vi "log analysis_gps.vi"() -> ()   [LabVIEW 2019] (continued)
\t", "INSPVAXA,USB3,0,48.0,FINESTEERING,2107,282547.800,02000000,471d,15824;INS_ALIGNMENT_COMPLETE,INS_RTKFIXED,37.37036979022,126.72474424169,11.9829,22.3000,0.0059,0.0077,0.0009,-0.935404379,-0.556069366,17.549298346,0.2070,0.1677,0.2732,0.0344,0.0343,0.0312,0.0907,0.0906,5.0042,0f000005,0*a5f569c8\n\t", "INSPVAXA,USB3,0,52.0,FINESTEERING,2107,282548.300,02000000,471d,15824;INS_ALIGNMENT_COMPLETE,INS_RTKFIXED,37.37036979009,126.72474424298,11.9833,22.3000,0.0058,0.0072,0.0008,-0.938145117,-0.556054082,17.551756735,0.2062,0.1674,0.2718,0.0344,0.0343,0.0312,0.0907,0.0906,5.0051,0f000005,0*c2e33c02\n\t", "INSPVAXA,USB3,0,50.5,FINESTEERING,2107,282549.300,02000000,471d,15824;INS_ALIGNMENT_COMPLETE,INS_RTKFIXED,37.37036979437,126.72474424171,11.9842,22.3000,0.0072,0.0058,0.0011,-0.941172709,-0.557765925,17.557830544,0.2056,0.1673,0.2705,0.0344,0.0343,0.0312,0.0907,0.0905,5.0063,0f000005,0*401534f2\n\t", "INSPVAXA,USB3,0,50.5,FINESTEERING,2107,282549.800,02000000,471d,15824;INS_ALIGNMENT_COMPLETE,INS_RTKFIXED,37.37037057498,126.72474454669,11.9842,22.3000,0.3344,0.1212,-0.0021,-0.779908756,-0.829652021,16.234479944,0.2056,0.1673,0.2705,0.0344,0.0343,0.0312,0.0907,0.0905,5.0063,0f000005,0*992e23a9\n\t", "INSPVAXA,USB3,0,48.5,FINESTEERING,2107,282550.300,02000000,471d,15824;INS_ALIGNMENT_COMPLETE,INS_RTKFIXED,37.37037180552,126.72474490570,11.9839,22.3000,0.3136,0.0717,0.0047,-0.762896217,-1.138555506,11.977754851,0.2091,0.1720,0.2750,0.0478,0.0529,0.0400,0.0942,0.0940,5.0079,0f000001,0*abd47146\n\t", "INSPVAXA,USB3,0,48.5,FINESTEERING,2107,282550.800,02000000,471d,15824;INS_ALIGNMENT_COMPLETE,INS_RTKFIXED,37.37037314462,126.72474521124,11.9825,22.3000,0.2954,0.0405,-0.0041,-0.725905831,-1.406758813,6.746591451,0.2091,0.1720,0.2750,0.0478,0.0529,0.0400,0.0942,0.0940,5.0079,0f000001,0*61668905\n\t", "INSPVAXA,USB3,0,51.5,FINESTEERING,2107,282551.300,02000000,471d,15824;INS_ALIGNMENT_COMPLETE,INS_RTKFIXED,37.37037450282,126.72474542954,11.9799,22.3000,0.2952,0.0275,0.0043,-0.582539496,-1.551817939,1.239321391,0.2194,0.1781,0.2846,0.0602,0.0670,0.0471,0.0975,0.0974,5.0042,0f000001,0*c43f8c5d\n\t", "INSPVAXA,USB3,0,51.5,FINESTEERING,2107,282551.800,02000000,471d,15824;INS_ALIGNMENT_COMPLETE,INS_RTKFIXED,37.37037589392,126.72474545445,11.9759,22.3000,0.2950,0.0095,-0.0088,-0.557235878,-1.675921373,356.051789382,0.2194,0.1781,0.2846,0.0602,0.0670,0.0471,0.0975,0.0974,5.0042,0f000001,0*a284eeef\n\t", "INSPVAXA,USB3,0,51.0,FINESTEERING,2107,282552.300,02000000,471d,15824;INS_ALIGNMENT_COMPLETE,INS_RTKFIXED,37.37037725637,126.72474539414,11.9729,22.3000,0.3193,-0.0395,-0.0058,-0.358098572,-1.586037546,351.118490428,0.2390,0.1944,0.2996,0.0720,0.0761,0.0531,0.1006,0.1005,4.9843,0f000001,0*9b67c117\n\t", "INSPVAXA,USB3,0,51.0,FINESTEERING,2107,282552.800,02000000,471d,15824;INS_ALIGNMENT_COMPLETE,INS_RTKFIXED,37.37037867024,126.72474521498,11.9693,22.3000,0.3100,-0.0524,0.0074,-0.558642327,-1.723684038,345.940999200,0.2390,0.1944,0.2996,0.0720,0.0761,0.0531,0.1006,0.1005,4.9843,0f000001,0*b237e03e\n\t", "INSPVAXA,USB3,0,50.0,FINESTEERING,2107,282553.800,02000000,471d,15824;INS_ALIGNMENT_COMPLETE,INS_RTKFIXED,37.37038133440,126.72474444492,11.9605,22.3000,0.3081,-0.0778,-0.0137,-0.440969194,-1.715960461,335.579383056,0.2674,0.2182,0.3198,0.0835,0.0827,0.0582,0.1031,0.1033,4.9481,0f000001,0*e6869deb\n\t", "INSPVAXA,USB3,0,50.5,FINESTEERING,2107,282554.300,02000000,471d,15824;INS_ALIGNMENT_COMPLETE,INS_RTKFIXED,37.37038260490,126.72474387942,11.9550,22.3000,0.2856,-0.1157,-0.0141,-0.305818210,-1.684904810,330.613449941,0.3015,0.2424,0.3440,0.0942,0.0885,0.0625,0.1050,0.1055,4.9097,0f000001,0*224ecce4\n\t", "INSPVAXA,USB3,0,50.5,FINESTEERING,2107,282554.800,02000000,471d,15824;INS_ALIGNMENT_COMPLETE,INS_RTKFIXED,37.37038381003,126.72474321955,11.9506,22.3000,0.2827,-0.1438,-0.0083,-0.269920364,-1.529846026,325.201495362,0.3015,0.2424,0.3440,0.0942,0.0885,0.0625,0.1050,0.1055,4.9097,0f000001,0*3a829f91\n\t", "INSPVAXA,USB3,0,50.0,FINESTEERING,2107,282555.300,02000000,471d,15824;INS_ALIGNMENT_COMPLETE,INS_RTKFIXED,37.37038496801,126.72474241807,11.9455,22.3000,0.2577,-0.2027,-0.0062,-0.202108415,-1.553117740,320.165911198,0.3366,0.2625,0.3706,0.1033,0.0925,0.0661,0.1060,0.1070,4.8793,0f000001,0*992111cd\n\t", "INSPVAXA,USB3,0,50.0,FINESTEERING,2107,282555.800,02000000,471d,15824;INS_ALIGNMENT_COMPLETE,INS_RTKFIXED,37.37038604879,126.72474155018,11.9405,22.3000,0.2577,-0.1938,-0.0290,0.085654909,-1.443333237,315.847452046,0.3366,0.2625,0.3706,0.1033,0.0925,0.0661,0.1060,0.1070,4.8793,0f000001,0*a6375ebe\n\t", "INSPVAXA,USB3,0,47.0,FINESTEERING,2107,282556.300,02000000,471d,15824;INS_ALIGNMENT_COMPLETE,INS_RTKFIXED,37.37038704857,126.72474062241,11.9355,22.3000,0.2432,-0.1774,-0.0062,0.142331168,-1.481321498,311.639962663,0.3685,0.2772,0.3979,0.1103,0.0957,0.0690,0.1063,0.1076,4.8620,0f000001,0*be30efa1\n\t", "INSPVAXA,USB3,0,47.0,FINESTEERING,2107,282556.800,02000000,471d,15824;INS_ALIGNMENT_COMPLETE,INS_RTKFIXED,37.37038792888,126.72473964017,11.9328,22.3000,0.2236,-0.2049,0.0022,0.167042140,-1.399079221,308.149842307,0.3685,0.2772,0.3979,0.1103,0.0957,0.0690,0.1063,0.1076,4.8620,0f000001,0*295fc098\n\t", "INSPVAXA,USB3,0,49.5,FINESTEERING,2107,282557.300,02000000,471d,15824;INS_ALIGNMENT_COMPLETE,INS_RTKFIXED,37.37038876743,126.72473857634,11.9284,22.3000,0.2199,-0.2115,-0.0007,0.223675096,-1.209289977,305.425052983,0.3945,0.2871,0.4244,0.1154,0.0985,0.0713,0.1059,0.1076,4.8550,0f000001,0*37184781\n\t", "INSPVAXA,USB3,0,49.5,FINESTEERING,2107,282557.800,02000000,471d,15824;INS_ALIGNMENT_COMPLETE,INS_RTKFIXED,37.37038956876,126.72473745081,11.9243,22.3000,0.2096,-0.2177,-0.0233,0.358750528,-1.202788361,303.229385124,0.3945,0.2871,0.4244,0.1154,0.0985,0.0713,0.1059,0.1076,4.8550,0f000001,0*8c1e375a\n\t", "INSPVAXA,USB3,0,50.5,FINESTEERING,2107,282558.300,02000000,471d,15824;INS_ALIGNMENT_COMPLETE,INS_RTKFIXED,37.37039033864,126.72473628263,11.9208,22.3000,0.2004,-0.2164,-0.0069,0.499556511,-1.306604746,301.526266622,0.4138,0.2933,0.4487,0.1187,0.1006,0.0729,0.1051,0.1069,4.8540,0f000001,0*451656bf\n\t", "INSPVAXA,USB3,0,50.5,FINESTEERING,2107,282558.800,02000000,471d,15824;INS_ALIGNMENT_COMPLETE,INS_RTKFIXED,37.37039107336,126.72473508379,11.9182,22.3000,0.1823,-0.2245,-0.0036,0.428634950,-1.459936721,300.166492995,0.4138,0.2933,0.4487,0.1187,0.1006,0.0729,0.1051,0.1069,4.8540,0f000001,0*b88ea368\n\t", "INSPVAXA,USB3,0,48.0,FINESTEERING,2107,282559.300,02000000,471d,15824;INS_ALIGNMENT_COMPLETE,INS_RTKFIXED,37.37039179926,126.72473381878,11.9163,22.3000,0.1950,-0.2202,-0.0095,0.298148012,-1.385671812,299.213023137,0.4272,0.2974,0.4700,0.1208,0.1020,0.0740,0.1041,0.1060,4.8546,0f000001,0*f3b6d2c4\n\t", "INSPVAXA,USB3,0,48.0,FINESTEERING,2107,282559.800,02000000,471d,15824;INS_ALIGNMENT_COMPLETE,INS_RTKFIXED,37.37039251718,126.72473255012,11.9132,22.3000,0.1990,-0.2202,-0.0184,0.279170037,-1.304746130,298.607357050,0.4272,0.2974,0.4700,0.1208,0.1020,0.0740,0.1041,0.1060,4.8546,0f000001,0*fce9781a\n\t", "DUALANTENNAHEADINGA,USB3,0,49.0,FINESTEERING,2107,282560.300,02000000,d426,15824;SOL_COMPUTED,L1_FLOAT,-1.000000000,246.253692627,40.984443665,0.0,360.000000000,180.000000000,\"631T\",16,4,4,4,04,00,20,00*676df0ad\n\t", "INSPVAXA,USB3,0,49.0,FINESTEERING,2107,282560.800,02000000,471d,15824;INS_ALIGNMENT_COMPLETE,INS_RTKFIXED,37.37039395485,126.72472993141,11.9024,22.3000,0.2031,-0.2330,-0.0176,0.316707422,-1.216731962,298.161405387,0.4358,0.3002,0.4880,0.1220,0.1029,0.0748,0.1029,0.1049,4.8545,0f000001,0*df5ab1e4\n\t", "DUALANTENNAHEADINGA,USB3,0,50.5,FINESTEERING,2107,282561.300,02000000,d426,15824;SOL_COMPUTED,L1_FLOAT,-1.000000000,334.919982910,-70.914154053,0.0,360.000000000,180.000000000,\"631T\",14,4,4,4,04,00,20,00*464ca699\n\t", "INSPVAXA,USB3,0,50.5,FINESTEERING,2107,282561.800,02000000,471d,15824;INS_ALIGNMENT_COMPLETE,INS_RTKFIXED,37.37039536755,126.72472721872,11.8937,22.3000,0.2015,-0.2233,-0.0217,0.095358091,-1.276712032,298.220729276,0.4412,0.3019,0.5026,0.1224,0.1030,0.0752,0.1017,0.1038,4.8530,0f000001,0*c4564f75\n\t", "DUALANTENNAHEADINGA,USB3,0,50.0,FINESTEERING,2107,282562.300,02000000,d426,15824;SOL_COMPUTED,L1_FLOAT,-1.000000000,248.535232544,17.692501068,0.0,360.000000000,180.000000000,\"631T\",15,4,4,4,04,00,20,00*bc5c3482\n\t", "INSPVAXA,USB3,0,50.0,FINESTEERING,2107,282562.800,02000000,471d,15824;INS_ALIGNMENT_COMPLETE,INS_RTKFIXED,37.37039678441,126.72472449457,11.8837,22.3000,0.2087,-0.2358,-0.0215,0.255454294,-1.083158063,298.402079920,0.4444,0.3029,0.5140,0.1223,0.1022,0.0754,0.1006,0.1028,4.8501,0f000001,0*9eae090a\n\t", "DUALANTENNAHEADINGA,USB3,0,51.0,FINESTEERING,2107,282563.300,02000000,d426,15824;SOL_COMPUTED,L1_FLOAT,-1.000000000,237.849975586,47.216407776,0.0,360.000000000,180.000000000,\"631T\",15,4,4,4,04,00,20,00*b09d8761\n\t", "DUALANTENNAHEADINGA,USB3,0,51.0,FINESTEERING,2107,282563.800,02000000,d426,15824;SOL_COMPUTED,L1_FLOAT,-1.000000000,239.350723267,46.591415405,0.0,360.000000000,180.000000000,\"631T\",14,4,4,4,04,00,20,00*f242e7bf\n\t", "DUALANTENNAHEADINGA,USB3,0,51.0,FINESTEERING,2107,282564.300,02000000,d426,15824;SOL_COMPUTED,L1_FLOAT,-1.000000000,238.787353516,46.982643127,0.0,360.000000000,180.000000000,\"631T\",14,4,4,4,04,00,20,00*054ac6ab\n\t", "DUALANTENNAHEADINGA,USB3,0,51.0,FINESTEERING,2107,282564.800,02000000,d426,15824;SOL_COMPUTED,L1_FLOAT,-1.000000000,245.656951904,39.742870331,0.0,360.000000000,180.000000000,\"631T\",14,4,4,4,04,00,20,00*f11cb885\n\t", "DUALANTENNAHEADINGA,USB3,0,52.0,FINESTEERING,2107,282565.300,02000000,d426,15824;SOL_COMPUTED,L1_FLOAT,-1.000000000,248.154891968,40.657573700,0.0,360.000000000,180.000000000,\"631T\",14,4,4,4,04,00,20,00*20192c08\n\t", "INSPVAXA,USB3,0,52.0,FINESTEERING,2107,282565.800,02000000,471d,15824;INS_ALIGNMENT_COMPLETE,INS_RTKFIXED,37.37040119345,126.72471623377,11.8630,22.3000,0.2075,-0.2604,-0.0264,0.476736901,-1.637367273,299.264508322,0.4468,0.3026,0.5333,0.1200,0.0984,0.0755,0.0985,0.1009,4.8387,0f000001,0*ff25f4bc\n\t", "INSPVAXA,USB3,0,51.5,FINESTEERING,2107,282566.300,02000000,471d,15824;INS_ALIGNMENT_COMPLETE,INS_RTKFIXED,37.37040195558,126.72471483727,11.8592,22.3000,0.1958,-0.2436,-0.0278,0.510354865,-1.544191392,299.414254294,0.4462,0.3017,0.5364,0.1190,0.0970,0.0755,0.0983,0.1007,4.8363,0f000001,0*b461588d\n\t", "INSPVAXA,USB3,0,51.5,FINESTEERING,2107,282566.800,02000000,471d,15824;INS_ALIGNMENT_COMPLETE,INS_RTKFIXED,37.37040269281,126.72471352564,11.8555,22.3000,0.1908,-0.2417,-0.0283,0.566870659,-1.494613883,299.549327154,0.4462,0.3017,0.5364,0.1190,0.0970,0.0755,0.0983,0.1007,4.8363,0f000001,0*0dca09ad\n\t", "DUALANTENNAHEADINGA,USB3,0,48.5,FINESTEERING,2107,282567.300,02000000,d426,15824;SOL_COMPUTED,L1_FLOAT,-1.000000000,255.600921631,36.764995575,0.0,360.000000000,180.000000000,\"631T\",14,4,4,4,04,00,20,00*5c98ac44\n\t", "DUALANTENNAHEADINGA,USB3,0,48.5,FINESTEERING,2107,282567.800,02000000,d426,15824;SOL_COMPUTED,L1_FLOAT,-1.000000000,256.974517822,34.665092468,0.0,360.000000000,180.000000000,\"631T\",13,4,4,4,04,00,20,00*958b7579\n\t", "DUALANTENNAHEADINGA,USB3,0,47.5,FINESTEERING,2107,282568.300,02000000,d426,15824;SOL_COMPUTED,L1_FLOAT,-1.000000000,267.947265625,0.986307323,0.0,360.000000000,180.000000000,\"631T\",15,4,4,4,04,00,20,00*84956e00\n\t", "DUALANTENNAHEADINGA,USB3,0,47.5,FINESTEERING,2107,282568.800,02000000,d426,15824;SOL_COMPUTED,L1_FLOAT,-1.000000000,262.026367188,14.068168640,0.0,360.000000000,180.000000000,\"631T\",16,4,4,4,04,00,20,00*8f55d343\n\t", "DUALANTENNAHEADINGA,USB3,0,50.0,FINESTEERING,2107,282569.300,02000000,d426,15824;SOL_COMPUTED,L1_FLOAT,-1.000000000,247.101364136,35.273887634,0.0,360.000000000,180.000000000,\"631T\",16,4,4,3,04,00,20,00*a64cde4f\n\t", "DUALANTENNAHEADINGA,USB3,0,50.0,FINESTEERING,2107,282569.800,02000000,d426,15824;SOL_COMPUTED,L1_FLOAT,-1.000000000,275.467193604,-13.373962402,0.0,360.000000000,180.000000000,\"631T\",15,4,4,4,04,00,20,00*431901e2\n\t", "DUALANTENNAHEADINGA,USB3,0,51.0,FINESTEERING,2107,282570.300,02000000,d426,15824;SOL_COMPUTED,L1_FLOAT,-1.000000000,299.108795166,-43.822387695,0.0,360.000000000,180.000000000,\"631T\",15,4,4,4,04,00,20,00*983d1a38\n\t", "DUALANTENNAHEADINGA,USB3,0,51.0,FINESTEERING,2107,282570.800,02000000,d426,15824;SOL_COMPUTED,L1_FLOAT,-1.000000000,300.479248047,-46.014068604,0.0,360.000000000,180.000000000,\"631T\",16,4,4,4,04,00,20,00*471f7ae7\n\t", "DUALANTENNAHEADINGA,USB3,0,50.5,FINESTEERING,2107,282571.300,02000000,d426,15824;SOL_COMPUTED,L1_FLOAT,-1.000000000,281.970092773,-22.784423828,0.0,360.000000000,180.000000000,\"631T\",16,4,4,4,04,00,20,00*6e1b1745\n\t", "DUALANTENNAHEADINGA,USB3,0,50.5,FINESTEERING,2107,282571.800,02000000,d426,15824;SOL_COMPUTED,L1_FLOAT,-1.000000000,280.621307373,-20.287109375,0.0,360.000000000,180.000000000,\"631T\",17,4,4,4,04,00,20,00*f2e1552e\n\t", "DUALANTENNAHEADINGA,USB3,0,50.5,FINESTEERING,2107,282572.300,02000000,d426,15824;SOL_COMPUTED,L1_FLOAT,-1.000000000,248.617050171,42.773250580,0.0,360.000000000,180.000000000,\"631T\",14,4,4,4,04,00,20,00*4f7db08e\n\t", "DUALANTENNAHEADINGA,USB3,0,50.5,FINESTEERING,2107,282572.800,02000000,d426,15824;SOL_COMPUTED,L1_FLOAT,-1.000000000,246.696640015,43.920532227,0.0,360.000000000,180.000000000,\"631T\",15,4,4,4,04,00,20,00*5d650678\n\t", "DUALANTENNAHEADINGA,USB3,0,47.0,FINESTEERING,2107,282573.300,02000000,d426,15824;SOL_COMPUTED,L1_FLOAT,-1.000000000,245.228240967,45.089698792,0.0,360.000000000,180.000000000,\"631T\",15,6,6,6,04,00,20,20*cc0e41c2\n\t", "DUALANTENNAHEADINGA,USB3,0,47.0,FINESTEERING,2107,282573.800,02000000,d426,15824;SOL_COMPUTED,L1_FLOAT,-1.000000000,244.818725586,44.919303894,0.0,360.000000000,180.000000000,\"631T\",15,6,6,6,04,00,20,20*3059716a\n\t", "DUALANTENNAHEADINGA,USB3,0,50.0,FINESTEERING,2107,282574.300,02000000,d426,15824;SOL_COMPUTED,L1_FLOAT,-1.000000000,234.880477905,50.460414886,0.0,146.039688110,120.522598267,\"631T\",15,6,6,6,04,00,20,20*c87e4a6e\n\t", "DUALANTENNAHEADINGA,USB3,0,50.0,FINESTEERING,2107,282574.800,02000000,d426,15824;SOL_COMPUTED,L1_FLOAT,-1.000000000,234.896896362,50.646526337,0.0,146.141387939,119.189933777,\"631T\",17,6,6,6,04,00,20,20*6b091558\n\t", "DUALANTENNAHEADINGA,USB3,0,47.0,FINESTEERING,2107,282575.300,02000000,d426,15824;SOL_COMPUTED,L1_FLOAT,-1.000000000,247.052993774,4.654780388,0.0,360.000000000,180.000000000,\"631T\",15,6,6,6,04,00,20,20*6353fb30\n\t", "DUALANTENNAHEADINGA,USB3,0,47.0,FINESTEERING,2107,282575.800,02000000,d426,15824;SOL_COMPUTED,L1_FLOAT,-1.000000000,247.398025513,2.300915241,0.0,360.000000000,180.000000000,\"631T\",16,6,6,6,04,00,20,20*f5a4c1cb\n\t", "DUALANTENNAHEADINGA,USB3,0,49.5,FINESTEERING,2107,282577.300,02000000,d426,15824;SOL_COMPUTED,L1_FLOAT,-1.000000000,245.373901367,33.916652679,0.0,360.000000000,180.000000000,\"631T\",14,4,4,4,04,00,20,00*102f57bf\n\t", "DUALANTENNAHEADINGA,USB3,0,49.5,FINESTEERING,2107,282577.800,02000000,d426,15824;SOL_COMPUTED,L1_FLOAT,-1.000000000,248.600692749,29.202283859,0.0,360.000000000,180.000000000,\"631T\",15,4,4,3,04,00,20,00*eaef8a59\n\t", "DUALANTENNAHEADINGA,USB3,0,50.0,FINESTEERING,2107,282578.300,02000000,d426,15824;SOL_COMPUTED,L1_FLOAT,-1.000000000,273.737609863,2.134390354,0.0,360.000000000,180.000000000,\"631T\",15,4,4,4,04,00,20,00*8bcfc7c6\n\t", "INSPVAXA,USB3,0,51.0,FINESTEERING,2107,282579.350,02000000,471d,15824;INS_ALIGNMENT_COMPLETE,INS_RTKFIXED,37.37041740707,126.72467743060,11.7862,22.3000,0.1031,-0.2921,-0.0179,0.173397794,-1.623675165,282.783174290,0.4573,0.2990,0.5534,0.1157,0.0933,0.0771,0.0996,0.1047,4.8395,0f000001,0*3f071db4\n\t", "DUALANTENNAHEADINGA,USB3,0,51.0,FINESTEERING,2107,282579.800,02000000,d426,15824;SOL_COMPUTED,L1_FLOAT,-1.000000000,253.552474976,36.318763733,0.0,360.000000000,180.000000000,\"631T\",12,4,4,4,04,00,20,00*83b3b49e\n\t", "DUALANTENNAHEADINGA,USB3,0,48.0,FINESTEERING,2107,282580.300,02000000,d426,15824;SOL_COMPUTED,L1_FLOAT,-1.000000000,276.287109375,16.184204102,0.0,360.000000000,180.000000000,\"631T\",13,4,4,4,04,00,20,00*58df2e4e\n\t", "INSPVAXA,USB3,0,48.0,FINESTEERING,2107,282580.850,02000000,471d,15824;INS_ALIGNMENT_COMPLETE,INS_RTKFIXED,37.37041861647,126.72467286120,11.7829,22.3000,0.1085,-0.2996,-0.0146,0.381599119,-1.778654518,281.769285798,0.4580,0.2991,0.5538,0.1158,0.0932,0.0771,0.0996,0.1049,4.8397,0f000001,0*ecbe1c22\n\t", "DUALANTENNAHEADINGA,USB3,0,49.0,FINESTEERING,2107,282581.800,02000000,d426,15824;SOL_COMPUTED,L1_FLOAT,-1.000000000,244.951904297,46.151142120,0.0,329.327331543,180.000000000,\"631T\",12,4,4,4,04,00,20,00*1c1834ad\n\t", "INSPVAXA,USB3,0,49.5,FINESTEERING,2107,282582.850,02000000,471d,15824;INS_ALIGNMENT_COMPLETE,INS_RTKFIXED,37.37042013529,126.72466675412,11.7738,22.3000,0.0889,-0.2912,-0.0157,0.137018151,-1.334468427,280.534881050,0.4569,0.2986,0.5535,0.1156,0.0931,0.0772,0.0995,0.1050,4.8407,0f000001,0*4cc88e7a\n\t", "DUALANTENNAHEADINGA,USB3,0,50.0,FINESTEERING,2107,282583.800,02000000,d426,15824;SOL_COMPUTED,L1_FLOAT,-1.000000000,298.425811768,-39.243469238,0.0,360.000000000,180.000000000,\"631T\",12,4,4,4,04,00,20,00*99234be7\n\t", "INSPVAXA,USB3,0,50.0,FINESTEERING,2107,282584.350,02000000,471d,15824;INS_ALIGNMENT_COMPLETE,INS_RTKFIXED,37.37042121578,126.72466218098,11.7682,22.3000,0.0908,-0.2905,-0.0097,0.228953863,-0.969786949,279.904204523,0.4542,0.2977,0.5520,0.1156,0.0930,0.0771,0.0995,0.1050,4.8423,0f000001,0*25d05607\n\t", "DUALANTENNAHEADINGA,USB3,0,50.0,FINESTEERING,2107,282584.800,02000000,d426,15824;SOL_COMPUTED,L1_FLOAT,-1.000000000,317.813751221,-55.080688477,0.0,360.000000000,180.000000000,\"631T\",14,4,4,4,04,00,20,00*482add9e\n\t", "DUALANTENNAHEADINGA,USB3,0,47.5,FINESTEERING,2107,282585.300,02008000,d426,15824;SOL_COMPUTED,L1_FLOAT,-1.000000000,279.031005859,-12.437835693,0.0,360.000000000,180.000000000,\"631T\",14,4,4,4,04,00,20,00*e33ff00b\n\t", "DUALANTENNAHEADINGA,USB3,0,47.5,FINESTEERING,2107,282585.800,02008000,d426,15824;SOL_COMPUTED,L1_FLOAT,-1.000000000,288.534484863,-28.210021973,0.0,360.000000000,180.000000000,\"631T\",14,4,4,4,04,00,20,00*75d90e5f\n\t", "DUALANTENNAHEADINGA,USB3,0,47.0,FINESTEERING,2107,282586.800,02008000,d426,15824;SOL_COMPUTED,L1_FLOAT,-1.000000000,299.638763428,-44.873535156,0.0,360.000000000,180.000000000,\"631T\",12,4,4,4,04,00,20,00*8433efc6\n\t", "DUALANTENNAHEADINGA,USB3,0,51.0,FINESTEERING,2107,282587.800,02008000,d426,15824;SOL_COMPUTED,L1_FLOAT,-1.000000000,274.837402344,7.455324173,0.0,360.000000000,180.000000000,\"631T\",12,4,4,4,04,00,20,00*d357c890\n\t", "INSPVAXA,USB3,0,53.0,FINESTEERING,2107,282588.350,02008000,471d,15824;INS_ALIGNMENT_COMPLETE,INS_RTKFIXED,37.37042392170,126.72464987629,11.7560,22.3000,0.0923,-0.2810,-0.0093,0.030566631,-0.932089530,279.991317390,0.4489,0.2966,0.5498,0.1150,0.0928,0.0771,0.0995,0.1049,4.8445,0f000001,0*cf0f29b3\n\t", "DUALANTENNAHEADINGA,USB3,0,53.0,FINESTEERING,2107,282588.800,02008000,d426,15824;SOL_COMPUTED,L1_FLOAT,-1.000000000,322.314697266,-55.526092529,0.0,360.000000000,180.000000000,\"631T\",12,4,4,4,04,00,20,00*c23a8009\n\t", "INSPVAXA,USB3,0,51.5,FINESTEERING,2107,282589.350,02000000,471d,15824;INS_ALIGNMENT_COMPLETE,INS_RTKFIXED,37.37042463832,126.72464679942,11.7536,22.3000,0.0961,-0.3116,-0.0160,0.320803902,-1.173970058,280.179307501,0.4487,0.2962,0.5495,0.1150,0.0928,0.0771,0.0995,0.1049,4.8450,0f000001,0*5f568f32\n\t", "INSPVAXA,USB3,0,51.5,FINESTEERING,2107,282589.850,02000000,471d,15824;INS_ALIGNMENT_COMPLETE,INS_RTKFIXED,37.37042500999,126.72464523335,11.7530,22.3000,0.0866,-0.2870,-0.0118,0.410270840,-1.158910418,280.360984304,0.4487,0.2962,0.5495,0.1150,0.0928,0.0771,0.0995,0.1049,4.8450,0f000001,0*cae4522e\n\t", "DUALANTENNAHEADINGA,USB3,0,50.5,FINESTEERING,2107,282590.300,02000000,d426,15824;INSUFFICIENT_OBS,NONE,-1.000000000,0.000000000,0.000000000,0.0,0.000000000,0.000000000,\"631T\",14,3,3,3,04,00,20,00*40a503c4\n\t", "INSPVAXA,USB3,0,49.0,FINESTEERING,2107,282591.350,02000000,471d,15824;INS_ALIGNMENT_COMPLETE,INS_RTKFIXED,37.37042612746,126.72464043128,11.7509,22.3000,0.1112,-0.3046,-0.0107,0.438593312,-1.353837387,280.922848312,0.4465,0.2958,0.5485,0.1145,0.0928,0.0771,0.0995,0.1048,4.8451,0f000001,0*466c5cb5\n\t", "INSPVAXA,USB3,0,48.0,FINESTEERING,2107,282592.350,02000000,471d,15824;INS_ALIGNMENT_COMPLETE,INS_RTKFIXED,37.37042693515,126.72463721970,11.7478,22.3000,0.1134,-0.2841,-0.0136,0.495116506,-1.748021922,281.445386324,0.4458,0.2955,0.5484,0.1143,0.0927,0.0771,0.0996,0.1048,4.8449,0f000001,0*7d422fc0\n\t", "INSPVAXA,USB3,0,51.5,FINESTEERING,2107,282593.350,02000000,471d,15824;INS_ALIGNMENT_COMPLETE,INS_RTKFIXED,37.37042777147,126.72463409939,11.7416,22.3000,0.1053,-0.2907,-0.0160,0.642644908,-1.933701573,282.530113202,0.4438,0.2953,0.5477,0.1141,0.0928,0.0771,0.0997,0.1048,4.8448,0f000001,0*602d795b\n\t", "INSPVAXA,USB3,0,51.5,FINESTEERING,2107,282593.850,02000000,471d,15824;INS_ALIGNMENT_COMPLETE,INS_RTKFIXED,37.37042819780,126.72463255781,11.7390,22.3000,0.0952,-0.2916,-0.0106,0.650646949,-1.972506612,283.259305122,0.4438,0.2953,0.5477,0.1141,0.0928,0.0771,0.0997,0.1048,4.8448,0f000001,0*d7827024\n\t", "INSPVAXA,USB3,0,49.5,FINESTEERING,2107,282594.350,02000000,471d,15824;INS_ALIGNMENT_COMPLETE,INS_RTKFIXED,37.37042864678,126.72463101246,11.7344,22.3000,0.0979,-0.2869,-0.0099,0.556878145,-1.878860029,284.055732763,0.4423,0.2949,0.5470,0.1139,0.0928,0.0770,0.0997,0.1048,4.8442,0f000001,0*f7248edf\n\t", "INSPVAXA,USB3,0,49.5,FINESTEERING,2107,282594.850,02000000,471d,15824;INS_ALIGNMENT_COMPLETE,INS_RTKFIXED,37.37042912060,126.72462947652,11.7289,22.3000,0.1303,-0.2985,-0.0065,0.456318200,-1.931761270,284.972124281,0.4423,0.2949,0.5470,0.1139,0.0928,0.0770,0.0997,0.1048,4.8442,0f000001,0*61f64e67\n\t", "INSPVAXA,USB3,0,48.5,FINESTEERING,2107,282595.350,02000000,471d,15824;INS_ALIGNMENT_COMPLETE,INS_RTKFIXED,37.37042961366,126.72462798098,11.7236,22.3000,0.1497,-0.2970,-0.0149,0.418327229,-1.868019582,285.752151928,0.4414,0.2947,0.5465,0.1139,0.0925,0.0770,0.0998,0.1049,4.8430,0f000001,0*1a617db7\n\t", "INSPVAXA,USB3,0,48.5,FINESTEERING,2107,282595.850,02000000,471d,15824;INS_ALIGNMENT_COMPLETE,INS_RTKFIXED,37.37043014219,126.72462646518,11.7180,22.3000,0.1392,-0.2900,-0.0231,0.427669167,-1.922456438,286.476446001,0.4414,0.2947,0.5465,0.1139,0.0925,0.0770,0.0998,0.1049,4.8430,0f000001,0*1a66d065\n\t", "INSPVAXA,USB3,0,50.5,FINESTEERING,2107,282596.350,02000000,471d,15824;INS_ALIGNMENT_COMPLETE,INS_RTKFIXED,37.37043069447,126.72462494509,11.7122,22.3000,0.1569,-0.2925,-0.0148,0.456002187,-2.188056466,287.205419298,0.4412,0.2946,0.5461,0.1139,0.0925,0.0770,0.0999,0.1050,4.8425,0f000001,0*15a09225\n\t", "INSPVAXA,USB3,0,50.5,FINESTEERING,2107,282596.850,02000000,471d,15824;INS_ALIGNMENT_COMPLETE,INS_RTKFIXED,37.37043125589,126.72462344785,11.7060,22.3000,0.1402,-0.2734,-0.0172,0.395468070,-2.411480135,287.743907623,0.4412,0.2946,0.5461,0.1139,0.0925,0.0770,0.0999,0.1050,4.8425,0f000001,0*9ae986ea\n\t", "INSPVAXA,USB3,0,49.0,FINESTEERING,2107,282597.350,02000000,471d,15824;INS_ALIGNMENT_COMPLETE,INS_RTKFIXED,37.37043180809,126.72462197460,11.7004,22.3000,0.1451,-0.2798,-0.0240,0.082189404,-2.342857619,288.211463548,0.4406,0.2943,0.5456,0.1138,0.0925,0.0770,0.1000,0.1050,4.8425,0f000001,0*a4baef99\n\t", "INSPVAXA,USB3,0,47.0,FINESTEERING,2107,282598.350,02000000,471d,15824;INS_ALIGNMENT_COMPLETE,INS_RTKFIXED,37.37043296335,126.72461906573,11.6872,22.3000,0.1639,-0.2709,-0.0144,0.075715172,-2.060890876,288.886128801,0.4401,0.2937,0.5452,0.1138,0.0925,0.0770,0.1001,0.1051,4.8435,0f000001,0*53c08aab\n\t", "INSPVAXA,USB3,0,47.0,FINESTEERING,2107,282598.850,02000000,471d,15824;INS_ALIGNMENT_COMPLETE,INS_RTKFIXED,37.37043354014,126.72461760390,11.6788,22.3000,0.1599,-0.2669,-0.0128,0.049311349,-2.026534390,289.114340802,0.4401,0.2937,0.5452,0.1138,0.0925,0.0770,0.1001,0.1051,4.8435,0f000001,0*6b176d5a\n\t", "INSPVAXA,USB3,0,48.5,FINESTEERING,2107,282599.350,02000000,471d,15824;INS_ALIGNMENT_COMPLETE,INS_RTKFIXED,37.37043410493,126.72461616545,11.6719,22.3000,0.1624,-0.2885,-0.0138,-0.156644949,-2.114929380,289.341942256,0.4397,0.2935,0.5448,0.1139,0.0926,0.0770,0.1001,0.1052,4.8449,0f000001,0*992413bc\n\t", "INSPVAXA,USB3,0,48.5,FINESTEERING,2107,282599.850,02000000,471d,15824;INS_ALIGNMENT_COMPLETE,INS_RTKFIXED,37.37043467790,126.72461472498,11.6664,22.3000,0.1607,-0.2703,-0.0125,-0.362948004,-2.133534264,289.548423016,0.4397,0.2935,0.5448,0.1139,0.0926,0.0770,0.1001,0.1052,4.8449,0f000001,0*c10a254e\n\t", "INSPVAXA,USB3,0,49.5,FINESTEERING,2107,282600.350,02000000,471d,15824;INS_ALIGNMENT_COMPLETE,INS_RTKFIXED,37.37043525953,126.72461325909,11.6615,22.3000,0.1615,-0.2803,-0.0148,-0.471431775,-2.267846962,289.732073791,0.4392,0.2934,0.5443,0.1138,0.0928,0.0769,0.1001,0.1052,4.8460,0f000001,0*36a380c0\n\t", "INSPVAXA,USB3,0,49.5,FINESTEERING,2107,282600.850,02000000,471d,15824;INS_ALIGNMENT_COMPLETE,INS_RTKFIXED,37.37043586783,126.72461175288,11.6568,22.3000,0.1684,-0.2866,-0.0132,-0.451303759,-2.269558677,289.856432048,0.4392,0.2934,0.5443,0.1138,0.0928,0.0769,0.1001,0.1052,4.8460,0f000001,0*3d745bd7\n\t", "INSPVAXA,USB3,0,47.5,FINESTEERING,2107,282601.350,02000000,471d,15824;INS_ALIGNMENT_COMPLETE,INS_RTKFIXED,37.37043647524,126.72461026809,11.6515,22.3000,0.1700,-0.2809,-0.0124,-0.328241253,-2.248777073,289.979230408,0.4390,0.2932,0.5439,0.1138,0.0927,0.0769,0.1000,0.1052,4.8467,0f000001,0*88c87769\n\t", "INSPVAXA,USB3,0,47.5,FINESTEERING,2107,282601.850,02000000,471d,15824;INS_ALIGNMENT_COMPLETE,INS_RTKFIXED,37.37043706474,126.72460883352,11.6472,22.3000,0.1674,-0.2631,-0.0107,-0.295120633,-2.255482926,290.118733293,0.4390,0.2932,0.5439,0.1138,0.0927,0.0769,0.1000,0.1052,4.8467,0f000001,0*60fbd16c\n\t", "INSPVAXA,USB3,0,49.5,FINESTEERING,2107,282602.350,02000000,471d,15824;INS_ALIGNMENT_COMPLETE,INS_RTKFIXED,37.37043766543,126.72460736241,11.6426,22.3000,0.1773,-0.2821,-0.0125,-0.322654423,-2.363199962,290.226882800,0.4388,0.2931,0.5437,0.1138,0.0926,0.0769,0.0999,0.1052,4.8468,0f000001,0*f3791758\n\t", "INSPVAXA,USB3,0,49.5,FINESTEERING,2107,282602.850,02000000,471d,15824;INS_ALIGNMENT_COMPLETE,INS_RTKFIXED,37.37043827005,126.72460590169,11.6385,22.3000,0.1821,-0.2724,-0.0121,-0.418675445,-2.261623622,290.351055865,0.4388,0.2931,0.5437,0.1138,0.0926,0.0769,0.0999,0.1052,4.8468,0f000001,0*204debac\n\t", "INSPVAXA,USB3,0,44.5,FINESTEERING,2107,282603.350,02000000,471d,15824;INS_ALIGNMENT_COMPLETE,INS_RTKFIXED,37.37043885036,126.72460451664,11.6355,22.3000,0.1725,-0.2572,-0.0117,-0.454843723,-2.160794151,290.461374575,0.4389,0.2930,0.5435,0.1139,0.0927,0.0769,0.0999,0.1052,4.8469,0f000001,0*fe35c8bb\n\t", "INSPVAXA,USB3,0,44.5,FINESTEERING,2107,282603.850,02000000,471d,15824;INS_ALIGNMENT_COMPLETE,INS_RTKFIXED,37.37043945299,126.72460307083,11.6317,22.3000,0.1803,-0.2729,-0.0125,-0.455229843,-2.077941582,290.572474787,0.4389,0.2930,0.5435,0.1139,0.0927,0.0769,0.0999,0.1052,4.8469,0f000001,0*cc614426\n\t", "INSPVAXA,USB3,0,48.5,FINESTEERING,2107,282604.350,02000000,471d,15824;INS_ALIGNMENT_COMPLETE,INS_RTKFIXED,37.37044007383,126.72460154659,11.6273,22.3000,0.1929,-0.2951,-0.0109,-0.392288663,-2.045966583,290.664646635,0.4392,0.2930,0.5434,0.1140,0.0926,0.0769,0.0998,0.1052,4.8464,0f000001,0*8e2e8e57\n\t", "INSPVAXA,USB3,0,46.0,FINESTEERING,2107,282605.850,02000000,471d,15824;INS_ALIGNMENT_COMPLETE,INS_RTKFIXED,37.37044182670,126.72459720127,11.6153,22.3000,0.1906,-0.2962,-0.0097,-0.601316831,-2.333994849,291.196527762,0.4394,0.2930,0.5433,0.1141,0.0926,0.0769,0.0997,0.1052,4.8458,0f000001,0*9a6d08c1\n\t", "INSPVAXA,USB3,0,47.0,FINESTEERING,2107,282606.350,02000000,471d,15824;INS_ALIGNMENT_COMPLETE,INS_RTKFIXED,37.37044241168,126.72459579253,11.6120,22.3000,0.1650,-0.2486,-0.0027,-0.608391314,-2.324818349,291.383905054,0.4412,0.2932,0.5437,0.1140,0.0926,0.0769,0.0996,0.1052,4.8446,0f000001,0*3d88472b\n\t", "INSPVAXA,USB3,0,47.0,FINESTEERING,2107,282606.850,02000000,471d,15824;INS_ALIGNMENT_COMPLETE,INS_RTKFIXED,37.37044299863,126.72459438872,11.6086,22.3000,0.1967,-0.2948,-0.0098,-0.716784784,-2.185835585,291.603581988,0.4412,0.2932,0.5437,0.1140,0.0926,0.0769,0.0996,0.1052,4.8446,0f000001,0*5390b691\n\t", "INSPVAXA,USB3,0,50.5,FINESTEERING,2107,282607.350,02000000,471d,15824;INS_ALIGNMENT_COMPLETE,INS_RTKFIXED,37.37044361320,126.72459293136,11.6060,22.3000,0.1791,-0.2405,0.0044,-0.624652897,-2.258872249,291.867019396,0.4427,0.2934,0.5443,0.1141,0.0925,0.0769,0.0996,0.1052,4.8437,0f000001,0*4de0af31\n\t", "INSPVAXA,USB3,0,50.5,FINESTEERING,2107,282607.850,02000000,471d,15824;INS_ALIGNMENT_COMPLETE,INS_RTKFIXED,37.37044423988,126.72459145739,11.6024,22.3000,0.1844,-0.2484,-0.0073,-0.519908618,-2.368148317,292.226693813,0.4427,0.2934,0.5443,0.1141,0.0925,0.0769,0.0996,0.1052,4.8437,0f000001,0*603a82db\n\t", "INSPVAXA,USB3,0,51.0,FINESTEERING,2107,282608.350,02000000,471d,15824;INS_ALIGNMENT_COMPLETE,INS_RTKFIXED,37.37044483752,126.72459005434,11.5979,22.3000,0.1715,-0.2554,-0.0122,-0.519117149,-2.380892114,292.717494679,0.4421,0.2933,0.5443,0.1142,0.0925,0.0769,0.0995,0.1051,4.8434,0f000001,0*764df120\n\t", "INSPVAXA,USB3,0,47.0,FINESTEERING,2107,282609.350,02000000,471d,15824;INS_ALIGNMENT_COMPLETE,INS_RTKFIXED,37.37044605652,126.72458722854,11.5885,22.3000,0.1663,-0.2764,-0.0069,-0.648305418,-2.537713416,293.939898101,0.4422,0.2933,0.5445,0.1140,0.0925,0.0769,0.0995,0.1051,4.8432,0f000001,0*830d3839\n\t", "INSPVAXA,USB3,0,49.0,FINESTEERING,2107,282610.350,02000000,471d,15824;INS_ALIGNMENT_COMPLETE,INS_RTKFIXED,37.37044732236,126.72458446831,11.5778,22.3000,0.1884,-0.2557,-0.0029,-0.876321406,-2.449391486,295.430567939,0.4418,0.2933,0.5445,0.1139,0.0924,0.0769,0.0995,0.1051,4.8434,0f000001,0*8a5ecd23\n\t", "INSPVAXA,USB3,0,48.5,FINESTEERING,2107,282611.350,02000000,471d,15824;INS_ALIGNMENT_COMPLETE,INS_RTKFIXED,37.37044865428,126.72458179844,11.5688,22.3000,0.1893,-0.2465,-0.0147,-0.836892789,-2.139837911,297.111108164,0.4413,0.2932,0.5444,0.1139,0.0924,0.0769,0.0995,0.1050,4.8437,0f000001,0*5c5081ba\n\t", "INSPVAXA,USB3,0,49.0,FINESTEERING,2107,282612.350,02000000,471d,15824;INS_ALIGNMENT_COMPLETE,INS_RTKFIXED,37.37045003475,126.72457914119,11.5590,22.3000,0.1912,-0.2423,-0.0135,-1.077738591,-1.947492637,298.710847895,0.4411,0.2932,0.5444,0.1142,0.0925,0.0769,0.0995,0.1050,4.8438,0f000001,0*1786ad92\n\t", "INSPVAXA,USB3,0,51.5,FINESTEERING,2107,282613.350,02000000,471d,15824;INS_ALIGNMENT_COMPLETE,INS_RTKFIXED,37.37045149851,126.72457646585,11.5487,22.3000,0.1950,-0.2536,-0.0123,-1.258648342,-2.137744772,299.825187137,0.4411,0.2932,0.5443,0.1140,0.0925,0.0769,0.0994,0.1050,4.8434,0f000001,0*52f4ee79\n\t", "INSPVAXA,USB3,0,46.0,FINESTEERING,2107,282614.350,02000000,471d,15824;INS_ALIGNMENT_COMPLETE,INS_RTKFIXED,37.37045301719,126.72457385904,11.5391,22.3000,0.2078,-0.2477,-0.0088,-1.293609252,-2.271198924,300.637369153,0.4405,0.2931,0.5441,0.1140,0.0925,0.0769,0.0994,0.1049,4.8428,0f000001,0*b4115fbd\n\t", "INSPVAXA,USB3,0,50.0,FINESTEERING,2107,282615.350,02000000,471d,15824;INS_ALIGNMENT_COMPLETE,INS_RTKFIXED,37.37045455007,126.72457134249,11.5267,22.3000,0.2142,-0.2258,-0.0244,-1.294164682,-1.774661927,301.229016667,0.4401,0.2931,0.5440,0.1144,0.0926,0.0769,0.0994,0.1049,4.8422,0f000001,0*3cd07d07\n\t", "INSPVAXA,USB3,0,50.5,FINESTEERING,2107,282620.350,02000000,471d,15824;INS_ALIGNMENT_COMPLETE,INS_RTKFIXED,37.37046253392,126.72455852077,11.4659,22.3000,0.2027,-0.2268,-0.0270,-1.031833865,-2.375437300,303.226270712,0.4405,0.2931,0.5444,0.1138,0.0928,0.0769,0.0992,0.1046,4.8369,0f000001,0*42a616f1\n\t", "INSPVAXA,USB3,0,49.5,FINESTEERING,2107,282623.850,02000000,471d,15824;INS_ALIGNMENT_COMPLETE,INS_RTKFIXED,37.37046800824,126.72454964821,11.4249,22.3000,0.1899,-0.2361,-0.0160,-1.285475051,-1.943866845,304.127219371,0.4404,0.2931,0.5447,0.1139,0.0925,0.0769,0.0992,0.1044,4.8359,0f000001,0*b0ab9613\n\t", "INSPVAXA,USB3,0,47.5,FINESTEERING,2107,282637.900,02008000,471d,15824;INS_ALIGNMENT_COMPLETE,INS_RTKFIXED,37.37049069819,126.72451409261,11.3482,22.3000,0.1872,-0.2201,-0.0214,-1.529619886,-2.288561964,301.270449465,0.4393,0.2929,0.5443,0.1132,0.0922,0.0769,0.0991,0.1040,4.8392,0f000001,0*31e93d15\n\t", "INSPVAXA,USB3,0,49.0,FINESTEERING,2107,282639.900,02000000,471d,15824;INS_ALIGNMENT_COMPLETE,INS_RTKFIXED,37.37049383425,126.72450900434,11.3318,22.3000,0.1967,-0.2325,-0.0119,-1.304734991,-1.946875629,300.584763179,0.4389,0.2928,0.5445,0.1134,0.0922,0.0769,0.0991,0.1040,4.8404,0f000001,0*b559a964\n\t", "INSPVAXA,USB3,0,51.5,FINESTEERING,2107,282642.900,02000000,471d,15824;INS_ALIGNMENT_COMPLETE,INS_RTKFIXED,37.37049844036,126.72450129803,11.3052,22.3000,0.1790,-0.2238,-0.0065,-1.283994704,-1.940797731,299.771183825,0.4397,0.2927,0.5445,0.1137,0.0922,0.0769,0.0991,0.1039,4.8409,0f000001,0*aafea47d\n\t", "INSPVAXA,USB3,0,50.0,FINESTEERING,2107,282643.400,02000000,471d,15824;INS_ALIGNMENT_COMPLETE,INS_RTKFIXED,37.37049919529,126.72450000565,11.2985,22.3000,0.1781,-0.2166,-0.0149,-1.239759750,-1.850856169,299.704406659,0.4403,0.2927,0.5448,0.1137,0.0922,0.0769,0.0991,0.1039,4.8403,0f000001,0*4cea9f21\n\t", "INSPVAXA,USB3,0,50.5,FINESTEERING,2107,282644.900,02000000,471d,15824;INS_ALIGNMENT_COMPLETE,INS_RTKFIXED,37.37050142661,126.72449611592,11.2793,22.3000,0.1856,-0.2171,-0.0219,-1.338634044,-1.925841589,299.522455316,0.4408,0.2928,0.5450,0.1137,0.0922,0.0769,0.0991,0.1039,4.8394,0f000001,0*5553cbbb\n\t", "INSPVAXA,USB3,0,50.5,FINESTEERING,2107,282647.400,02000000,471d,15824;INS_ALIGNMENT_COMPLETE,INS_RTKFIXED,37.37050513933,126.72448960666,11.2512,22.3000,0.1984,-0.2298,-0.0285,-1.166556084,-1.704562940,299.605783810,0.4451,0.2932,0.5473,0.1143,0.0922,0.0771,0.0990,0.1039,4.8365,0f000001,0*2668bb94\n\t", "INSPVAXA,USB3,0,50.5,FINESTEERING,2107,282647.900,02000000,471d,15824;INS_ALIGNMENT_COMPLETE,INS_RTKFIXED,37.37050588895,126.72448827979,11.2460,22.3000,0.1904,-0.2211,-0.0266,-1.200661987,-1.937489399,299.682292940,0.4451,0.2932,0.5473,0.1143,0.0922,0.0771,0.0990,0.1039,4.8365,0f000001,0*df8b46cf\n\t", "INSPVAXA,USB3,0,50.0,FINESTEERING,2107,282649.900,02000000,471d,15824;INS_ALIGNMENT_COMPLETE,INS_RTKFIXED,37.37050893925,126.72448297158,11.2267,22.3000,0.1903,-0.2023,-0.0241,-0.768669991,-2.369260824,300.015949522,0.4461,0.2933,0.5487,0.1140,0.0923,0.0771,0.0990,0.1039,4.8348,0f000001,0*dea76ac5\n\t", "INSPVAXA,USB3,0,51.5,FINESTEERING,2107,282650.400,02000000,471d,15824;INS_ALIGNMENT_COMPLETE,INS_RTKFIXED,37.37050972480,126.72448163294,11.2213,22.3000,0.2048,-0.2320,-0.0314,-0.685414349,-2.106294081,300.095837477,0.4453,0.2931,0.5488,0.1140,0.0923,0.0771,0.0990,0.1038,4.8348,0f000001,0*243c57b4\n\t", "INSPVAXA,USB3,0,45.5,FINESTEERING,2107,282651.900,02000000,471d,15824;INS_ALIGNMENT_COMPLETE,INS_RTKFIXED,37.37051201880,126.72447778068,11.2078,22.3000,0.1916,-0.2205,-0.0248,-0.576530745,-1.861777705,300.300269268,0.4449,0.2931,0.5488,0.1139,0.0923,0.0771,0.0990,0.1038,4.8347,0f000001,0*af26017a\n\t", "INSPVAXA,USB3,0,51.5,FINESTEERING,2107,282653.900,02000000,471d,15824;INS_ALIGNMENT_COMPLETE,INS_RTKFIXED,37.37051509510,126.72447251131,11.1945,22.3000,0.1929,-0.2150,-0.0150,-0.802596336,-1.882184040,300.662762095,0.4446,0.2931,0.5493,0.1139,0.0923,0.0771,0.0991,0.1038,4.8344,0f000001,0*a735d545\n\t", "INSPVAXA,USB3,0,49.5,FINESTEERING,2107,282654.400,02000000,471d,15824;INS_ALIGNMENT_COMPLETE,INS_RTKFIXED,37.37051584618,126.72447125334,11.1924,22.3000,0.2065,-0.2512,-0.0226,-0.731158373,-1.931164870,300.740729096,0.4441,0.2931,0.5492,0.1141,0.0922,0.0771,0.0991,0.1038,4.8345,0f000001,0*6bec4445\n\t", "INSPVAXA,USB3,0,49.5,FINESTEERING,2107,282655.400,02000000,471d,15824;INS_ALIGNMENT_COMPLETE,INS_RTKFIXED,37.37051739369,126.72446865376,11.1860,22.3000,0.1911,-0.2128,-0.0292,-0.646981835,-2.105939863,300.753498708,0.4442,0.2930,0.5492,0.1138,0.0923,0.0771,0.0991,0.1038,4.8345,0f000001,0*03f7e14e\n\t", "INSPVAXA,USB3,0,49.5,FINESTEERING,2107,282655.900,02000000,471d,15824;INS_ALIGNMENT_COMPLETE,INS_RTKFIXED,37.37051816950,126.72446734615,11.1828,22.3000,0.1941,-0.2176,-0.0241,-0.579402849,-2.122031776,300.745538986,0.4442,0.2930,0.5492,0.1138,0.0923,0.0771,0.0991,0.1038,4.8345,0f000001,0*dfac7fa4\n\t", "INSPVAXA,USB3,0,50.0,FINESTEERING,2107,282656.400,02000000,471d,15824;INS_ALIGNMENT_COMPLETE,INS_RTKFIXED,37.37051892940,126.72446603782,11.1784,22.3000,0.1975,-0.2201,-0.0250,-0.527531498,-2.256977557,300.738893590,0.4437,0.2930,0.5489,0.1139,0.0923,0.0771,0.0991,0.1038,4.8347,0f000001,0*858cd015\n\t", "INSPVAXA,USB3,0,50.0,FINESTEERING,2107,282657.400,02000000,471d,15824;INS_ALIGNMENT_COMPLETE,INS_RTKFIXED,37.37052044371,126.72446344968,11.1671,22.3000,0.1932,-0.2068,-0.0116,-0.414783465,-2.317412537,300.721707080,0.4433,0.2930,0.5487,0.1138,0.0923,0.0770,0.0992,0.1038,4.8350,0f000001,0*72bd9a4b\n\t", "INSPVAXA,USB3,0,50.0,FINESTEERING,2107,282657.900,02000000,471d,15824;INS_ALIGNMENT_COMPLETE,INS_RTKFIXED,37.37052121955,126.72446213298,11.1620,22.3000,0.2017,-0.2233,-0.0206,-0.308273301,-2.524902992,300.688892174,0.4433,0.2930,0.5487,0.1138,0.0923,0.0770,0.0992,0.1038,4.8350,0f000001,0*cf92748e\n\t", "INSPVAXA,USB3,0,48.0,FINESTEERING,2107,282658.400,02000000,471d,15824;INS_ALIGNMENT_COMPLETE,INS_RTKFIXED,37.37052197544,126.72446081424,11.1558,22.3000,0.2035,-0.2219,-0.0181,-0.328078319,-2.511940655,300.637576073,0.4425,0.2930,0.5482,0.1137,0.0923,0.0770,0.0992,0.1038,4.8355,0f000001,0*376bbad4\n\t", "INSPVAXA,USB3,0,48.0,FINESTEERING,2107,282658.900,02000000,471d,15824;INS_ALIGNMENT_COMPLETE,INS_RTKFIXED,37.37052272730,126.72445951727,11.1488,22.3000,0.1942,-0.2149,-0.0164,-0.313220820,-2.516289447,300.678904806,0.4425,0.2930,0.5482,0.1137,0.0923,0.0770,0.0992,0.1038,4.8355,0f000001,0*e2928abf\n\t", "INSPVAXA,USB3,0,50.5,FINESTEERING,2107,282660.400,02000000,471d,15824;INS_ALIGNMENT_COMPLETE,INS_RTKFIXED,37.37052497375,126.72445559407,11.1294,22.3000,0.1977,-0.2195,-0.0225,-0.387313372,-2.271618505,300.730077872,0.4409,0.2929,0.5472,0.1136,0.0922,0.0770,0.0992,0.1038,4.8370,0f000001,0*69452c97\n\t", "INSPVAXA,USB3,0,50.5,FINESTEERING,2107,282660.900,02000000,471d,15824;INS_ALIGNMENT_COMPLETE,INS_RTKFIXED,37.37052574047,126.72445427382,11.1237,22.3000,0.1897,-0.2035,-0.0252,-0.381842817,-2.256778592,300.817684769,0.4409,0.2929,0.5472,0.1136,0.0922,0.0770,0.0992,0.1038,4.8370,0f000001,0*d5bdd052\n\t", "INSPVAXA,USB3,0,49.5,FINESTEERING,2107,282661.400,02000000,471d,15824;INS_ALIGNMENT_COMPLETE,INS_RTKFIXED,37.37052651141,126.72445295109,11.1180,22.3000,0.1959,-0.2165,-0.0224,-0.305806610,-2.215640419,300.881180775,0.4410,0.2930,0.5471,0.1137,0.0922,0.0770,0.0993,0.1038,4.8381,0f000001,0*01198745\n\t", "INSPVAXA,USB3,0,49.5,FINESTEERING,2107,282661.900,02000000,471d,15824;INS_ALIGNMENT_COMPLETE,INS_RTKFIXED,37.37052725992,126.72445165392,11.1131,22.3000,0.1958,-0.2218,-0.0300,-0.421587704,-2.162878960,300.913228762,0.4410,0.2930,0.5471,0.1137,0.0922,0.0770,0.0993,0.1038,4.8381,0f000001,0*8e192d49\n\t", "INSPVAXA,USB3,0,52.0,FINESTEERING,2107,282662.400,02000000,471d,15824;INS_ALIGNMENT_COMPLETE,INS_RTKFIXED,37.37052801675,126.72445034380,11.1087,22.3000,0.1896,-0.2102,-0.0176,-0.535002925,-2.143447457,300.990757797,0.4412,0.2930,0.5470,0.1137,0.0922,0.0770,0.0993,0.1038,4.8391,0f000001,0*8c4251fb\n\t", "INSPVAXA,USB3,0,52.0,FINESTEERING,2107,282662.900,02000000,471d,15824;INS_ALIGNMENT_COMPLETE,INS_RTKFIXED,37.37052880342,126.72444898642,11.1040,22.3000,0.1905,-0.2142,-0.0217,-0.575840592,-2.161837706,301.070112972,0.4412,0.2930,0.5470,0.1137,0.0922,0.0770,0.0993,0.1038,4.8391,0f000001,0*2ee126c6\n\t", "INSPVAXA,USB3,0,49.0,FINESTEERING,2107,282663.400,02000000,471d,15824;INS_ALIGNMENT_COMPLETE,INS_RTKFIXED,37.37052954535,126.72444770805,11.0993,22.3000,0.2098,-0.2404,-0.0214,-0.590246803,-1.901325753,301.153923627,0.4417,0.2932,0.5470,0.1139,0.0924,0.0770,0.0993,0.1038,4.8402,0f000001,0*c89c711f\n\t", "DUALANTENNAHEADINGA,USB3,0,49.0,FINESTEERING,2107,282663.900,02000000,d426,15824;SOL_COMPUTED,L1_FLOAT,-1.000000000,333.457733154,12.245697021,0.0,360.000000000,180.000000000,\"631T\",15,5,5,5,04,00,20,20*8b83e92e\n\t", "INSPVAXA,USB3,0,45.5,FINESTEERING,2107,282664.400,02000000,471d,15824;INS_ALIGNMENT_COMPLETE,
